vi "DIAdem Process Report Request.vi"(8 "error in (no error)":errorcluster, 10 "DIAdem Queue":T1, 11 "DIAdem Reference":T3) -> (0 "error out":errorcluster, 1 "Done?":bool, 2 "Output":string, 3 "dup DIAdem Reference":T3)   [LabVIEW 2011]
uses:
  <vilib>/ExportToExcel/DIAdem Reference.ctl
  DIAdem Daemon Queue.ctl
  DIAdem Daemon Script Type.ctl
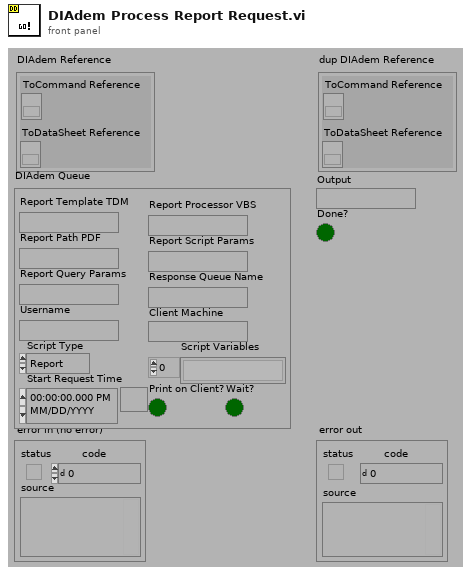
[diagram p1: front panel]
types:
  T1 = typedef "DIAdem Daemon Queue.ctl" = cluster{"Report Template TDM":path, "Report Processor VBS":path, "Report Path PDF":path, "Report Script Params":string, "Username":string, "Script Type":T2, "Report Query Params":string, "Client Machine":string, "Print on Client?":bool, "Response Queue Name":string, "Script Variables":string[], "Start Request Time":timestamp, "Wait?":bool}
  T2 = typedef "DIAdem Daemon Script Type.ctl" = enum16{"Report", "Query", "Script", "Datasheet", "Append", "Restart", "Stop"}
  T3 = typedef "DIAdem Reference.ctl" = cluster{"ToCommand Reference":refnum<k7>, "ToDataSheet Reference":refnum<k7>}
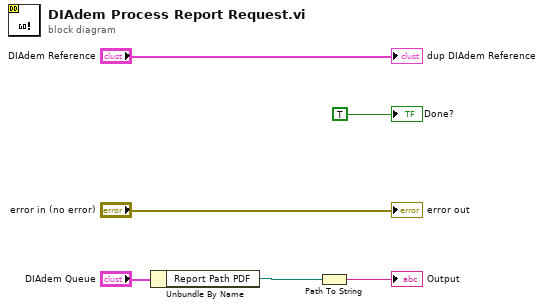
[diagram p0: block diagram]
diagram:
  n1 = Unbundle By Name("DIAdem Queue") -> ("Report Path PDF"=w3:path)
  n2 = Path To String(path=w3) -> (string=→"Output":string)
  "error out" <- "error in (no error)"
  "dup DIAdem Reference" <- "DIAdem Reference"
  "Done?" <- TRUE
